vi "Scan TU Number.vi"(10 "Lookup Path":path) -> (0 "OK?":bool, 2 "TU Number Out":string)   [LabVIEW 2024, in "LVarex.lvlib"]
uses:
  LVarex.lvlib
panel:
  out "First Scan?":bool
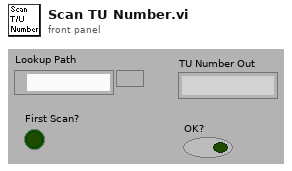
[diagram p1: front panel]
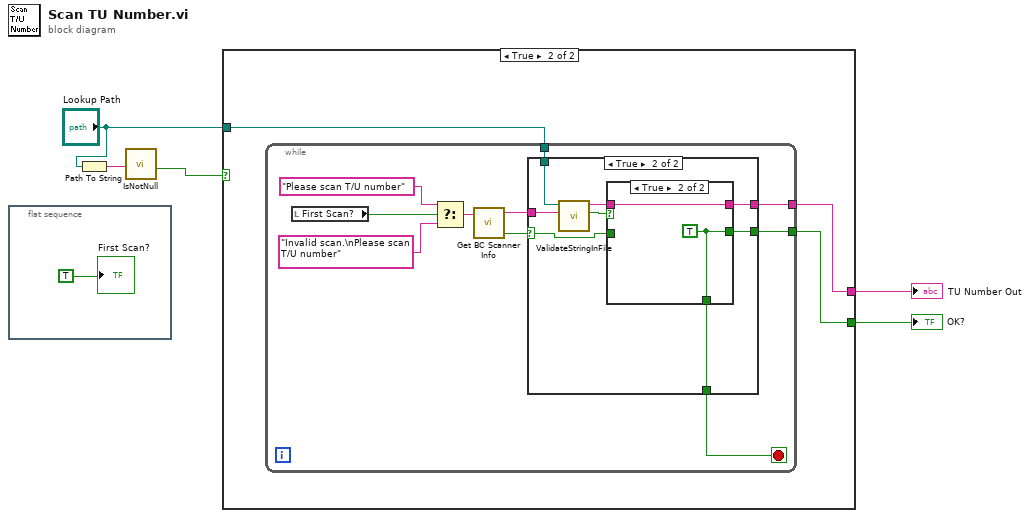
[diagram p0: block diagram]
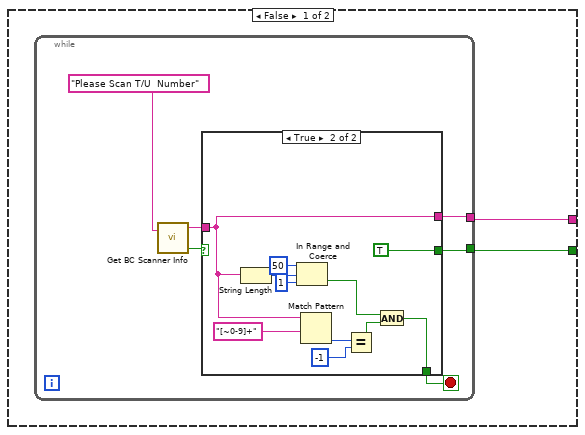
[diagram p2: hidden frame]
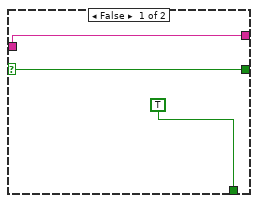
[diagram p3: hidden frame]
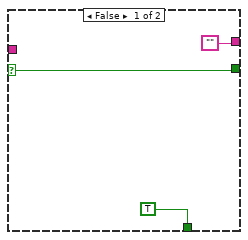
[diagram p4: hidden frame]
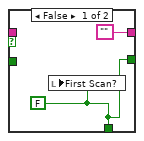
[diagram p5: hidden frame]
diagram:
  n1 = flat-sequence {
    frame #0 {
      "First Scan?" <- TRUE
    }
  }
  n2 = Path To String(path="Lookup Path") -> (string=w2:string)
  n3 = call "IsNotNull.vi"("String In"=w2) -> ("Boolean Out"=w1:bool)  [unwired: 10 in]
  n4 = case shown="True" w1 {
    tunnel: [w8 w30] -> w5
    tunnel: [w7 w29] -> w4
    tunnel: "Lookup Path" -> [_ w31]
    frame False {
      n5 = while {
        tunnel: [w12] -> w7
        tunnel: [w11] -> w8
        stop <- w10 stop-if-true
        n6 = call "Get BC Scanner Info.vi"("Prompt"="Please Scan T/U  Number") -> ("Info Out"=w9:string, "OK"=w13:bool)  [unwired: 2 in]
        n7 = case shown="True" w13 {
          selector: w13 -> [w17 _]
          tunnel: [w17 TRUE] -> w12
          tunnel: w9 -> [w16 w24]
          tunnel: [w16 w24] -> w11
          tunnel: [TRUE w18] -> w10
          frame False {
          }
          frame True {
            n8 = String Length(string=w24) -> (length=w27:i32)
            n9 = In Range and Coerce(upper limit=50, x=w27, lower limit=1) -> (In Range?=w19:bool)  [unwired: 1 out]
            n10 = Match Pattern(string=w24, regular expression="[~0-9]+") -> (offset past match=w22:i32)  [unwired: 1 in, 3 out]
            n11 = Equal?(x=w22, y=-1 ("x")) -> (x = y?=w20:bool)
            n12 = And(x=w19, y=w20) -> (x .and. y?=w18:bool)
          }
        }
      }
    }
    frame True {
      n13 = while {
        tunnel: w31 -> [w35]
        tunnel: [w34] -> w30
        tunnel: [w33] -> w29
        stop <- w32 stop-if-true
        n14 = local read "First Scan?"() -> (w39:bool)
        n15 = Select(t="Please scan T/U number", s=w39, f="Invalid scan.\nPlease scan T/U number") -> (s? t:f=w38:string)
        n16 = call "Get BC Scanner Info.vi"("Prompt"=w38) -> ("Info Out"=w37:string, "OK"=w36:bool)  [unwired: 2 in]
        n17 = case shown="True" w36 {
          selector: w36 -> [w42 w47]
          tunnel: w37 -> [_ w52]
          tunnel: w35 -> [_ w51]
          tunnel: ["" w48] -> w34
          tunnel: [w42 w46] -> w33
          tunnel: [TRUE w45] -> w32
          frame False {
          }
          frame True {
            n18 = call "ValidateStringInFile.vi"("String to find"=w52, "Path In"=w51) -> ("String Found"=w49:bool, "String Out"=w50:string)  [unwired: 7 in, 1 out]
            n19 = case shown="True" w49 {
              tunnel: w50 -> [_ w56]
              tunnel: ["" w56] -> w48
              tunnel: w47 -> [_ _]
              tunnel: [w54 w55] -> w46
              tunnel: [w54 w55] -> w45
              frame False {
                w54 = FALSE
                n20 = local write "First Scan?"(w54) -> ()
              }
              frame True {
                w55 = TRUE
              }
            }
          }
        }
      }
    }
  }
  "TU Number Out" <- w5
  "OK?" <- w4
